vi "odd and even.vi"() -> ()   [LabVIEW 2018]
panel:
  in  "Elements":dbl[](array[numeric])
  out "Even no":dbl[](array[numeric])
  out "Odd no":dbl[](array[numeric])
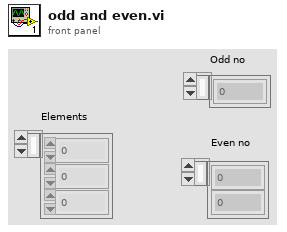
[diagram p1: front panel]
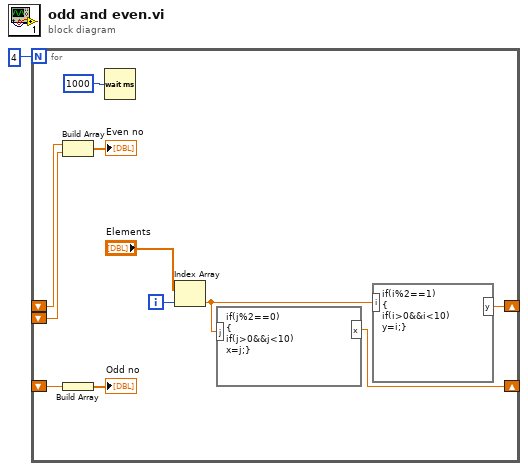
[diagram p0: block diagram]
diagram:
  n1 = for {
    N: 4 -> [_]
    shift-right: [w8] -> _
    shift-left: _ -> [w10]
    shift-right: [w9] -> _
    shift-left: _ -> [w7]
    shift-left: _ -> [w6]
    i -> [w5]
    n2 = Build Array(w7, w6) -> (→"Even no":dbl[])
    n3 = Build Array(w10) -> (→"Odd no":dbl[])
    n4 = Wait (ms)(milliseconds to wait=u32 1000) -> ()  [unwired: 1 out]
    n5 = Index Array(array="Elements", index=w5) -> (element=w11:dbl)
    n6 = formula code="if(j%2==0)\n{\nif(j>0&&j<10)\nx=j;}"("j"=w11) -> ("x"=w8:dbl)
    n7 = formula code="if(i%2==1)\n{\nif(i>0&&i<10)\ny=i;}"("i"=w11) -> ("y"=w9:dbl)
  }
